vi "Coherent cmnd pst-proc L1 (direct).vi"(7 "Coherent laser commands L1":T1=enum."Set Command", 8 "error in (no error)":errorcluster, 10 "Response String":string, 11 "Command String":string) -> (0 "error out":errorcluster, 1 "Response String":string, 2 "Response Validated ?":bool, 3 "trimmed string":string, 4 "Command String":string)   [LabVIEW 2020]
uses:
  Type defs/Coherent comms control.ctl
panel:
  out "offset past match":i32
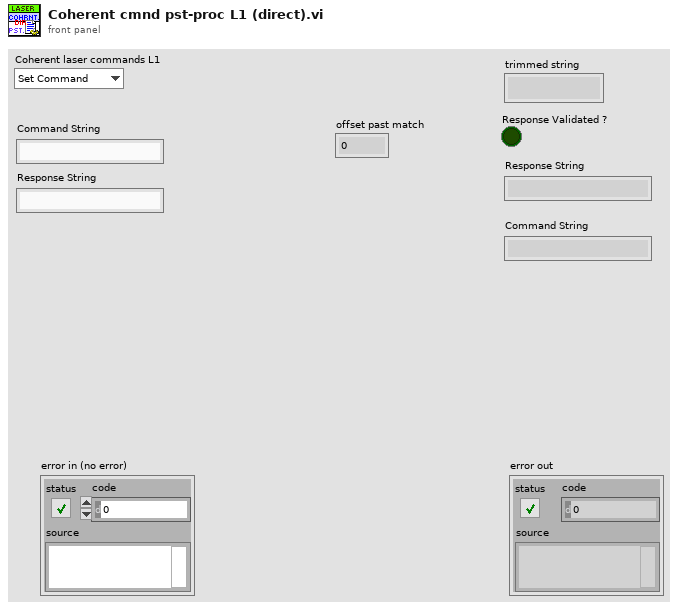
[diagram p1: front panel]
types:
  T1 = typedef "Coherent comms control.ctl" = enum16{"Initialise", "Get Command", "Set Command", "Clear Buffer", "Close"}
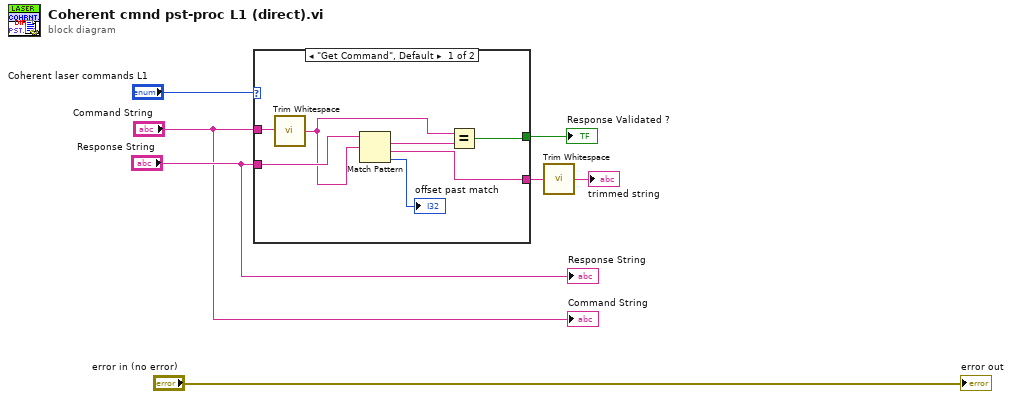
[diagram p0: block diagram]
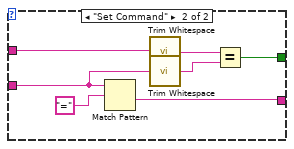
[diagram p2: hidden frame]
diagram:
  n1 = case shown="\"Get Command\", Default" "Coherent laser commands L1" {
    tunnel: "Response String" -> [w14 w15]
    tunnel: "Command String" -> [w9 w17]
    tunnel: [w13 w20] -> w3
    tunnel: [w10 w18] -> w2
    frame "Get Command", Default {
      n2 = call <vilib>:"Trim Whitespace.vi"("string"=w9) -> ("trimmed string"=w8:string)  [unwired: 1 in]
      n3 = Match Pattern(string=w14, regular expression=w8) -> (match substring=w11:string, after substring=w13:string, offset past match=→"offset past match":i32)  [unwired: 1 in, 1 out]
      n4 = Equal?(x=w8, y=w11) -> (x = y?=w10:bool)
    }
    frame "Set Command" {
      n5 = Match Pattern(string=w15, regular expression="=") -> (after substring=w20:string)  [unwired: 1 in, 3 out]
      n6 = call <vilib>:"Trim Whitespace.vi"("string"=w17) -> ("trimmed string"=w16:string)  [unwired: 1 in]
      n7 = call <vilib>:"Trim Whitespace.vi"("string"=w15) -> ("trimmed string"=w19:string)  [unwired: 1 in]
      n8 = Equal?(x=w16, y=w19) -> (x = y?=w18:bool)
    }
  }
  "Response Validated ?" <- w2
  n9 = call <vilib>:"Trim Whitespace.vi"("string"=w3) -> ("trimmed string"=→"trimmed string":string)  [unwired: 1 in]
  "Response String" <- "Response String"
  "error out" <- "error in (no error)"
  "Command String" <- "Command String"
